vi "CHECK Sv(SubVI).vi"(9 "B3    in":bool, 10 "B2    in":bool, 11 "B1   in":bool) -> (3 "Numeric":dbl)   [LabVIEW 2018]
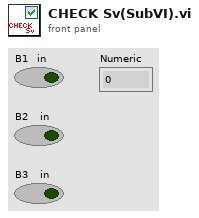
[diagram p1: front panel]
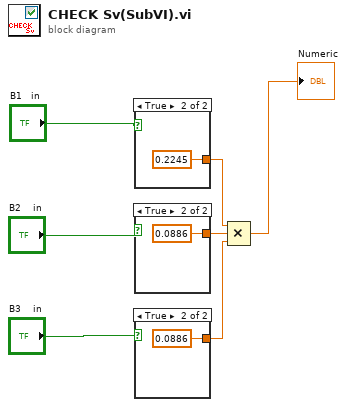
[diagram p0: block diagram]
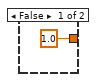
[diagram p2: hidden frame]
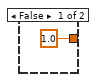
[diagram p3: hidden frame]
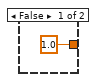
[diagram p4: hidden frame]
diagram:
  n1 = case shown="True" "B1   in" {
    tunnel: [1.0 0.2245] -> w2
    frame False {
    }
    frame True {
    }
  }
  n2 = case shown="True" "B2    in" {
    tunnel: [1.0 0.0886] -> w3
    frame False {
    }
    frame True {
    }
  }
  n3 = case shown="True" "B3    in" {
    tunnel: [1.0 0.0886] -> w4
    frame False {
    }
    frame True {
    }
  }
  n4 = Compound Arithmetic op=MULTIPLY(w2, w3, w4) -> (→"Numeric":dbl)
